vi "Testresizetobiggestdecor.vi"   [LabVIEW 2022 SP3]
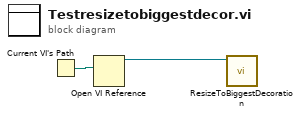
[diagram p0: block diagram]
diagram:
  n1 = Current VI's Path() -> (path=w2:path)
  n2 = Open VI Reference(vi path=w2) -> (vi reference=w1:refnum<vi>)  [unwired: 5 in, 1 out]
  n3 = call "ResizeToBiggestDecoration.vi"("VI in"=w1) -> ()  [unwired: 10 in, 1 out]
